vi "Decimal Degrees from dddmm.mmm.vi"(1 "Hemisphere Letter":string, 2 "Degrees String":string) -> (0 "Decimal Degrees":dbl format="%#_12g")   [LabVIEW 2010]
doc: "Give this VI decimal degrees in the format [d]ddmm.mmmmm and a hemisphere letter (N,E,S,W) and it will return decimal degrees with the correct sign."
uses:
  <vilib>/regexp/Match Regular Expression.xnode
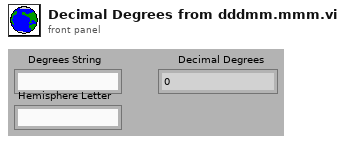
[diagram p1: front panel]
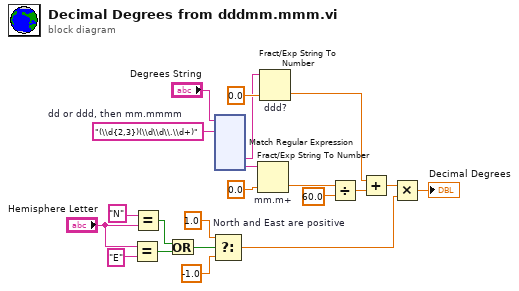
[diagram p0: block diagram]
diagram:
  w3 = "(\\d{2,3})(\\d\\d\\.\\d+)"  # dd or ddd, then mm.mmmm
  n1 = Equal?(x="Hemisphere Letter", y="E") -> (x = y?=w14:bool)
  n2 = Equal?(x="N" ("y"), y="Hemisphere Letter") -> (x = y?=w13:bool)
  n3 = Or(x=w13, y=w14) -> (x .or. y?=w12:bool)
  n4 = Select "North and East are positive"(t=1.0, s=w12, f=-1.0) -> (s? t:f=w7:dbl)
  n5 = xnode "Match Regular Expression"("input string"="Degrees String", "regular expression"=w3) -> ("submatch 1"=w2:string, "submatch 2"=w1:string)  [unwired: 2 in, 7 out]
  n6 = Fract/Exp String To Number "mm.m+"(string=w1, default (0 dbl)=0.0 ("x")) -> (number=w19:dbl)  [unwired: 3 out]
  n7 = Fract/Exp String To Number "ddd?"(string=w2, default (0 dbl)=0.0 ("x")) -> (number=w20:dbl)  [unwired: 3 out]
  n8 = Divide(x=w19, y=60.0) -> (x/y=w18:dbl)
  n9 = Add(x=w20, y=w18) -> (x+y=w5:dbl)
  n10 = Multiply(x=w5, y=w7) -> (x*y=→"Decimal Degrees":dbl)
